vi "Plot Camera Color Data.vi"(0 "Angle and color code of Green Buoys":dbl[][](array[numeric]), 5 "Angle and color code of Red Buoys":dbl[][](array[numeric])=[[-33.38976812661023, 1.0], [-12.98490982701509, 1.0]], 7 "Angle and color code of Yellow Buoys":dbl[][](array[numeric])=[[-33.38976812661023, 1.0], [-12.98490982701509, 1.0]], 9 "Angle and color code of Blue Buoys":dbl[][](array[numeric])=[[-33.38976812661023, 1.0], [-12.98490982701509, 1.0]], 11 "Angle and color code of Orange Buoys":dbl[][](array[numeric])=[[-33.38976812661023, 1.0], [-12.98490982701509, 1.0]]) -> (1 "Green Distance":dbl[](array[numeric]), 2 "Red Distance":dbl[](array[numeric]), 3 "Yellow Distance":dbl[](array[numeric]), 8 "XY Graph":cluster{dbl[], dbl[]}[](graph), 12 "Blue Distance":dbl[](array[numeric]), 13 "Orange Distance":dbl[](array[numeric]))   [LabVIEW 2018]
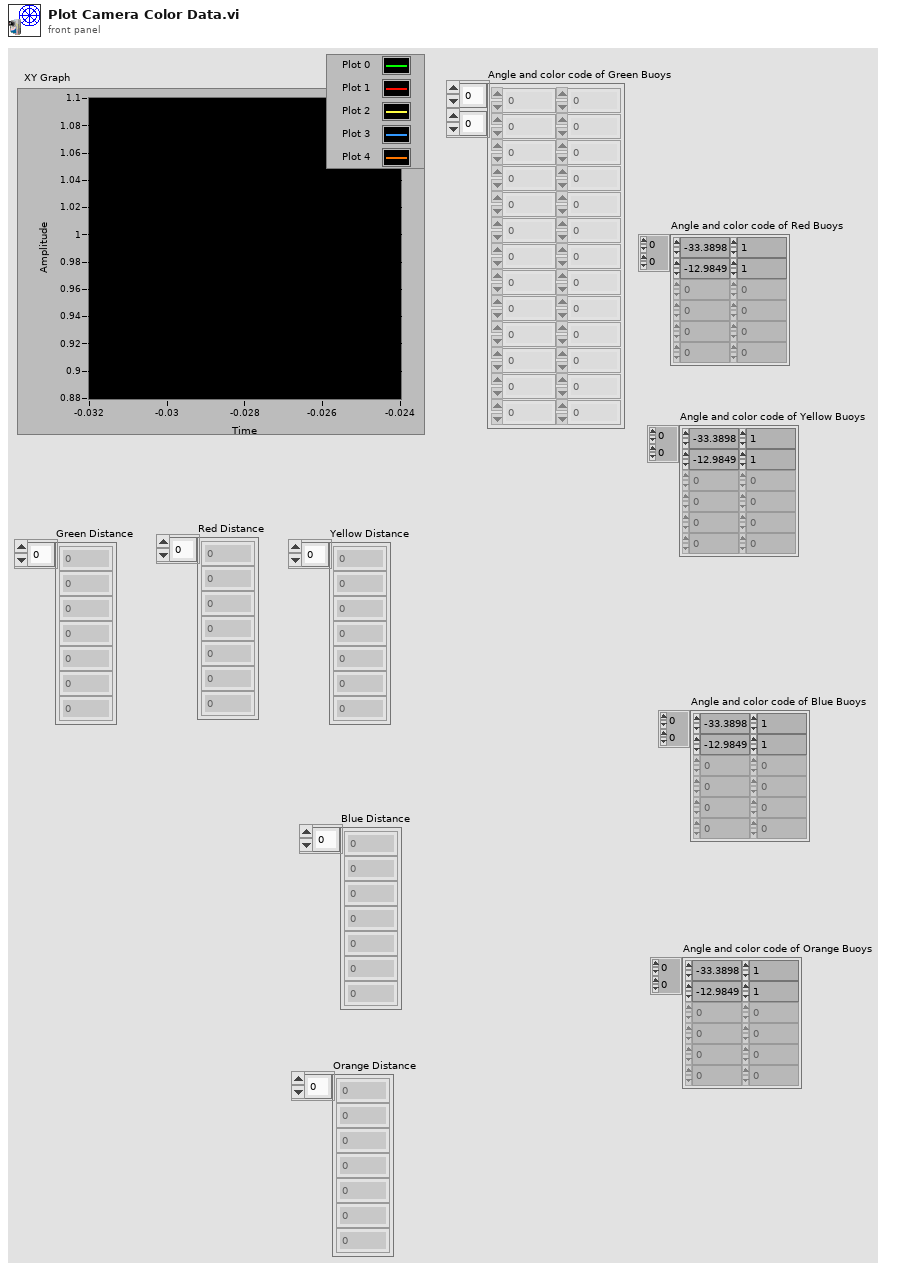
[diagram p1: front panel]
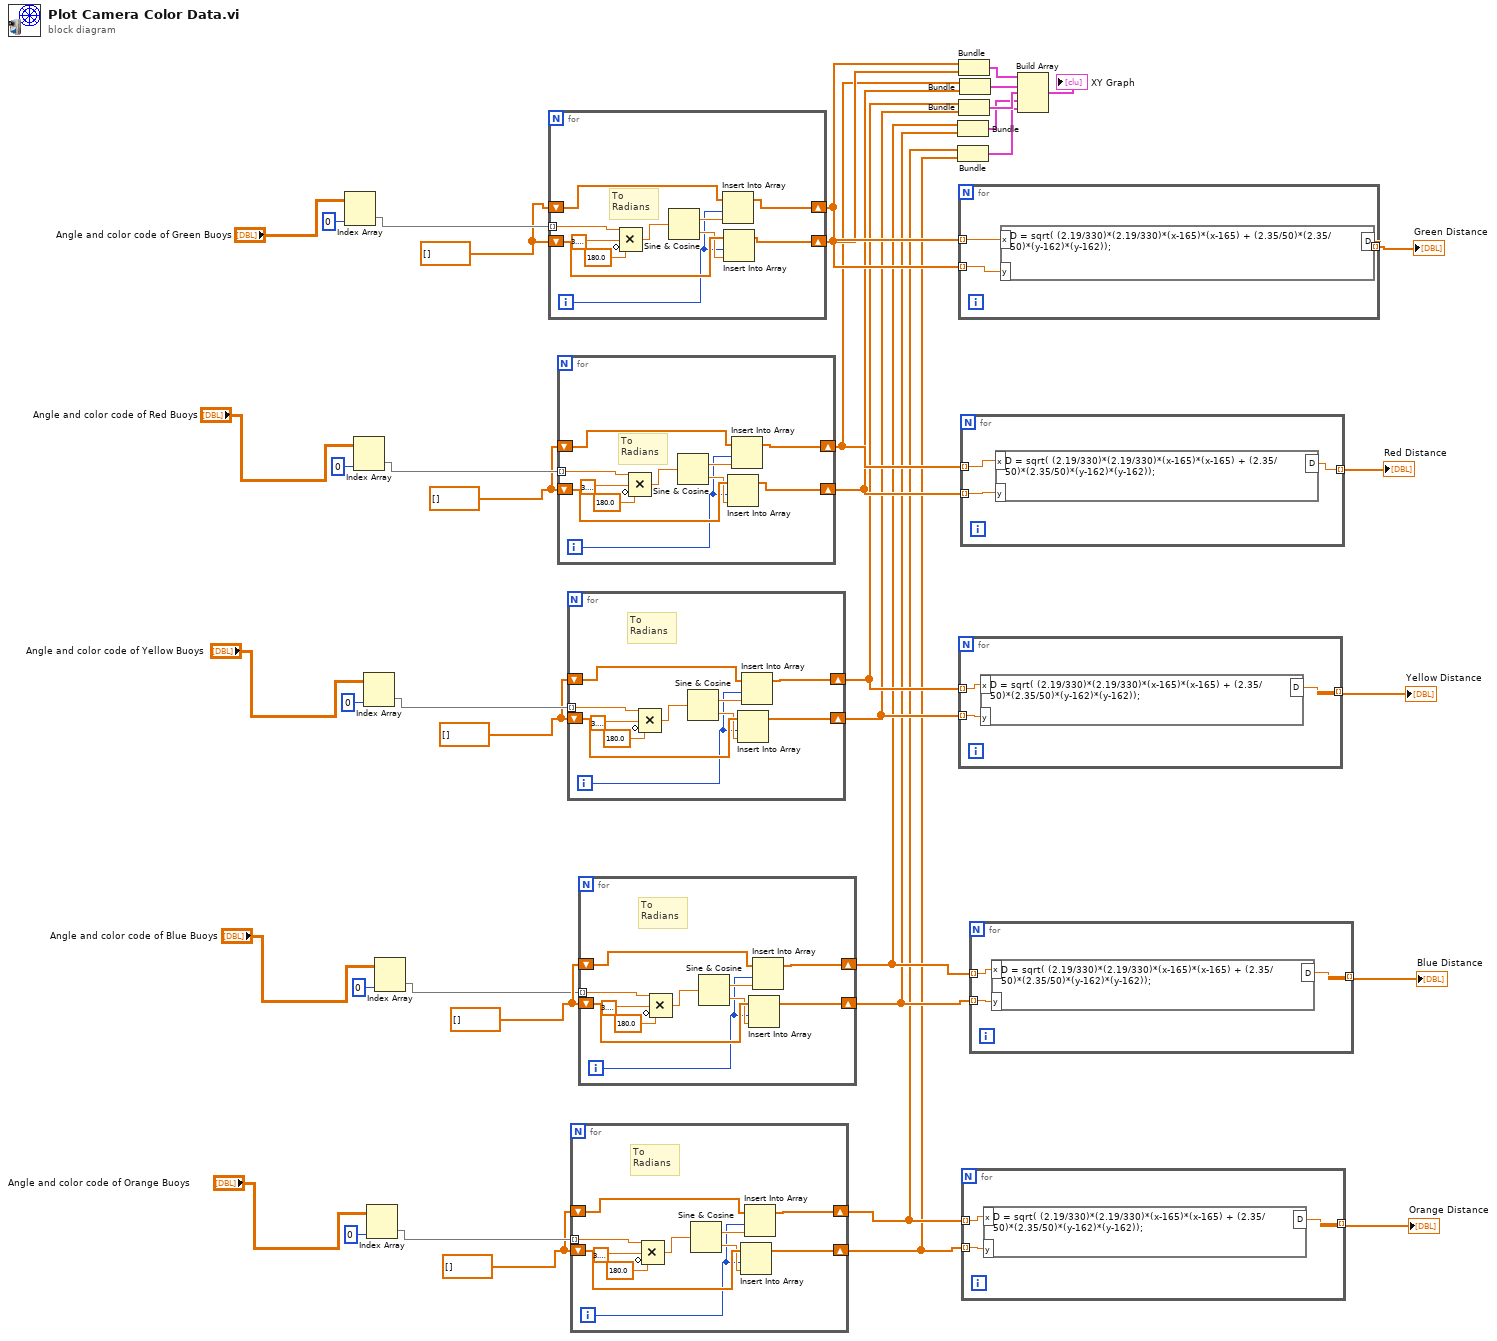
[diagram p0: block diagram]
diagram:
  w8 = dbl[] []
  w15 = dbl[] []
  w30 = dbl[] []
  w38 = dbl[] []
  w34 = dbl[] []
  n1 = Index Array(array="Angle and color code of Green Buoys", index (col)=0 ("disabled index (col)")) -> (element=w37:dbl[])  [unwired: 1 in]
  n2 = Index Array(array="Angle and color code of Red Buoys", index (col)=0 ("disabled index (col)")) -> (element=w40:dbl[])  [unwired: 1 in]
  n3 = Index Array(array="Angle and color code of Yellow Buoys", index (col)=0 ("disabled index (col)")) -> (element=w32:dbl[])  [unwired: 1 in]
  n4 = Index Array(array="Angle and color code of Orange Buoys", index (col)=0 ("disabled index (col)")) -> (element=w10:dbl[])  [unwired: 1 in]
  n5 = Index Array(array="Angle and color code of Blue Buoys", index (col)=0 ("disabled index (col)")) -> (element=w13:dbl[])  [unwired: 1 in]
  n6 = for {
    tunnel: w37 -> [w49] mode=indexing
    shift-right: [w42] -> w29
    shift-left: w34 -> [w48]
    shift-right: [w44] -> w28
    shift-left: w34 -> [w46]
    i -> [w43]
    # "To\nRadians"
    n7 = Compound Arithmetic op=MULTIPLY(w49, 3.141592653589793, invert 180.0 ("value")) -> (w50:dbl)
    n8 = Sine & Cosine(0:w50) -> (1:w47:dbl, 2:w45:dbl)
    n9 = Insert Into Array(array=w48, index=w43, new element=w47) -> (w42:dbl[])
    n10 = Insert Into Array(array=w46, index=w43, new element=w45) -> (w44:dbl[])
  }
  n11 = for {
    tunnel: w40 -> [w60] mode=indexing
    shift-right: [w58] -> w27
    shift-left: w38 -> [w59]
    shift-right: [w54] -> w26
    shift-left: w38 -> [w56]
    i -> [w53]
    # "To\nRadians"
    n12 = Compound Arithmetic op=MULTIPLY(w60, 3.141592653589793, invert 180.0 ("value")) -> (w61:dbl)
    n13 = Sine & Cosine(0:w61) -> (1:w57:dbl, 2:w55:dbl)
    n14 = Insert Into Array(array=w56, index=w53, new element=w55) -> (w54:dbl[])
    n15 = Insert Into Array(array=w59, index=w53, new element=w57) -> (w58:dbl[])
  }
  n16 = for {
    tunnel: w32 -> [w71] mode=indexing
    shift-right: [w69] -> w25
    shift-left: w30 -> [w70]
    shift-right: [w65] -> w24
    shift-left: w30 -> [w67]
    i -> [w64]
    # "To\nRadians"
    n17 = Compound Arithmetic op=MULTIPLY(w71, 3.141592653589793, invert 180.0 ("value")) -> (w72:dbl)
    n18 = Sine & Cosine(0:w72) -> (1:w68:dbl, 2:w66:dbl)
    n19 = Insert Into Array(array=w67, index=w64, new element=w66) -> (w65:dbl[])
    n20 = Insert Into Array(array=w70, index=w64, new element=w68) -> (w69:dbl[])
  }
  n21 = for {
    tunnel: w10 -> [w82] mode=indexing
    shift-right: [w80] -> w2
    shift-left: w8 -> [w81]
    shift-right: [w76] -> w1
    shift-left: w8 -> [w78]
    i -> [w75]
    # "To\nRadians"
    n22 = Compound Arithmetic op=MULTIPLY(w82, 3.141592653589793, invert 180.0 ("value")) -> (w83:dbl)
    n23 = Sine & Cosine(0:w83) -> (1:w79:dbl, 2:w77:dbl)
    n24 = Insert Into Array(array=w78, index=w75, new element=w77) -> (w76:dbl[])
    n25 = Insert Into Array(array=w81, index=w75, new element=w79) -> (w80:dbl[])
  }
  n26 = for {
    tunnel: w13 -> [w93] mode=indexing
    shift-right: [w91] -> w4
    shift-left: w15 -> [w92]
    shift-right: [w87] -> w3
    shift-left: w15 -> [w89]
    i -> [w86]
    # "To\nRadians"
    n27 = Compound Arithmetic op=MULTIPLY(w93, 3.141592653589793, invert 180.0 ("value")) -> (w94:dbl)
    n28 = Sine & Cosine(0:w94) -> (1:w90:dbl, 2:w88:dbl)
    n29 = Insert Into Array(array=w89, index=w86, new element=w88) -> (w87:dbl[])
    n30 = Insert Into Array(array=w92, index=w86, new element=w90) -> (w91:dbl[])
  }
  n31 = Bundle(w4, w3) -> (w6:cluster{dbl[], dbl[]})  [unwired: 1 in]
  n32 = Bundle(w2, w1) -> (w5:cluster{dbl[], dbl[]})  [unwired: 1 in]
  n33 = Bundle(w29, w28) -> (w23:cluster{dbl[], dbl[]})  [unwired: 1 in]
  n34 = Bundle(w25, w24) -> (w22:cluster{dbl[], dbl[]})  [unwired: 1 in]
  n35 = for {
    tunnel: w29 -> [w99] mode=indexing
    tunnel: w28 -> [w98] mode=indexing
    tunnel: [w97] -> w18 mode=indexing
    n36 = formula code="D = sqrt( (2.19/330)*(2.19/330)*(x-165)*(x-165) + (2.35/50)*(2.35/50)*(y-162)*(y-162));"("x"=w99, "y"=w98) -> ("D"=w97:dbl)
  }
  "Green Distance" <- w18
  n37 = for {
    tunnel: w25 -> [w102] mode=indexing
    tunnel: w24 -> [w101] mode=indexing
    tunnel: [w100] -> w19 mode=indexing
    n38 = formula code="D = sqrt( (2.19/330)*(2.19/330)*(x-165)*(x-165) + (2.35/50)*(2.35/50)*(y-162)*(y-162));"("x"=w102, "y"=w101) -> ("D"=w100:dbl)
  }
  "Yellow Distance" <- w19
  n39 = Bundle(w27, w26) -> (w21:cluster{dbl[], dbl[]})  [unwired: 1 in]
  n40 = for {
    tunnel: w27 -> [w105] mode=indexing
    tunnel: w26 -> [w104] mode=indexing
    tunnel: [w103] -> w17 mode=indexing
    n41 = formula code="D = sqrt( (2.19/330)*(2.19/330)*(x-165)*(x-165) + (2.35/50)*(2.35/50)*(y-162)*(y-162));"("x"=w105, "y"=w104) -> ("D"=w103:dbl)
  }
  "Red Distance" <- w17
  n42 = for {
    tunnel: w2 -> [w108] mode=indexing
    tunnel: w1 -> [w107] mode=indexing
    tunnel: [w106] -> w7 mode=indexing
    n43 = formula code="D = sqrt( (2.19/330)*(2.19/330)*(x-165)*(x-165) + (2.35/50)*(2.35/50)*(y-162)*(y-162));"("x"=w108, "y"=w107) -> ("D"=w106:dbl)
  }
  "Orange Distance" <- w7
  n44 = for {
    tunnel: w4 -> [w111] mode=indexing
    tunnel: w3 -> [w110] mode=indexing
    tunnel: [w109] -> w16 mode=indexing
    n45 = formula code="D = sqrt( (2.19/330)*(2.19/330)*(x-165)*(x-165) + (2.35/50)*(2.35/50)*(y-162)*(y-162));"("x"=w111, "y"=w110) -> ("D"=w109:dbl)
  }
  "Blue Distance" <- w16
  n46 = Build Array(w23, w21, w22, w6, w5) -> (→"XY Graph":cluster{dbl[], dbl[]}[])
